vi "ClusterControls.vi"() -> ()   [LabVIEW 2016, in "test_ValueSignal.lvlib"]
uses:
  test_ValueSignal.lvlib
  Helper/HelperVI1.vi
  main/apis/Stimulus/ValueSignalByPathString.vi
  main/apis/Assert/AssertControlValueByPathString.vi
  <vilib>/addons/_JKI Toolkits/Caraya/classes/Assert/Assert Equal Value_Variant.vi
  <vilib>/addons/_JKI Toolkits/Caraya/classes/Assert/Assert.lvclass
  <vilib>/addons/_JKI Toolkits/Caraya/classes/Test/Test.lvclass
panel:
  out "error out":errorcluster
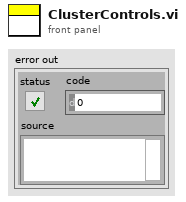
[diagram p1: front panel]
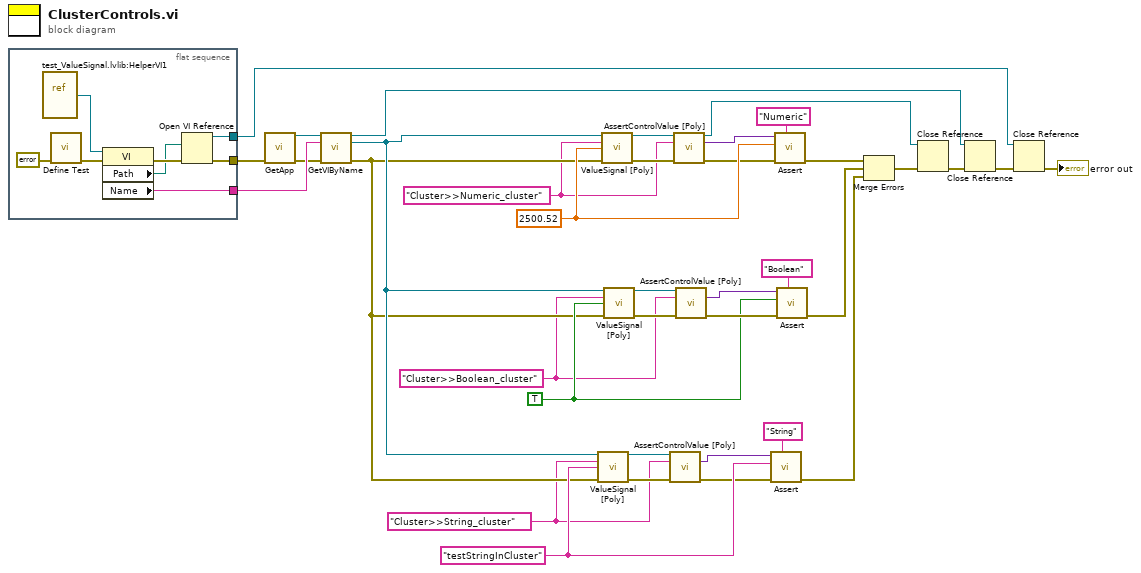
[diagram p0: block diagram]
diagram:
  w1 = "Cluster>>String_cluster"
  w2 = "Cluster>>Boolean_cluster"
  w3 = "Cluster>>Numeric_cluster"
  w17 = "testStringInCluster"
  w20 = TRUE
  w29 = 2500.52
  n1 = flat-sequence {
    tunnel: [w41] -> w32
    tunnel: [w40] -> w34
    tunnel: [w38] -> w31
    frame #0 {
      n2 = vi-ref "test_ValueSignal.lvlib:HelperVI1.vi"() -> (w43:refnum<vi>)
      n3 = call <vilib>:"Define Test.vi"("error in (no error)"=errorcluster {"status"=FALSE, "code"=0, "source"=""}) -> ("error out"=w44:errorcluster)  [unwired: 10 in]
      n4 = property on="Property Node" class="VI"(reference=w43, error in=w44) -> (error out=w42:errorcluster, "Path"=w39:path, "Name"=w38:string)  [unwired: 1 out]
      n5 = Open VI Reference(vi path=w39, error in (no error)=w42) -> (vi reference=w40:refnum<vi>, error out=w41:errorcluster)  [unwired: 4 in]
    }
  }
  n6 = call "GetApp.vi"("error in (no error)"=w32) -> ("Application Ref"=w33:refnum<vi>, "error out"=w30:errorcluster)  [unwired: 13 in]
  n7 = call "GetVIByName.vi"("Application Ref in"=w33, "VI Name"=w31, "error in (no error)"=w30) -> ("Application Ref out"=w5:refnum<vi>, "VI Reference"=w12:refnum<vi>, "error out"=w4:errorcluster)  [unwired: 10 in]
  n8 = call-poly "ValueSignal [Poly].vi"("VI Reference In"=w12, "Control Name"=w1, "Value (Signaling)"=w17, "error in"=w4) -> ("VI Reference Out"=w16:refnum<vi>, "error out"=w15:errorcluster)  [unwired: 10 in]
  n9 = call-poly "ValueSignal [Poly].vi"("VI Reference In"=w12, "Control Name"=w3, "Value (Signaling)"=w29, "error in"=w4) -> ("VI Reference Out"=w28:refnum<vi>, "error out"=w27:errorcluster)  [unwired: 10 in]
  n10 = call-poly "ValueSignal [Poly].vi"("VI Reference In"=w12, "Control Name"=w2, "Value (Signaling)"=w20, "error in"=w4) -> ("VI Reference Out"=w21:refnum<vi>, "error out"=w22:errorcluster)  [unwired: 10 in]
  n11 = call-poly "AssertControlValue [Poly].vi"("VI Reference In"=w16, "Control Name"=w1, "error in"=w15) -> ("Value"=w13:variant, "error out"=w14:errorcluster)  [unwired: 10 in, 1 out]
  n12 = call-poly "AssertControlValue [Poly].vi"("VI Reference In"=w28, "Control Name"=w3, "error in"=w27) -> ("VI Reference Out"=w7:refnum<vi>, "Value"=w25:variant, "error out"=w26:errorcluster)  [unwired: 10 in]
  n13 = call-poly "AssertControlValue [Poly].vi"("VI Reference In"=w21, "Control Name"=w2, "error in"=w22) -> ("Value"=w24:variant, "error out"=w23:errorcluster)  [unwired: 10 in, 1 out]
  n14 = call-poly <vilib>:"Assert.vi"("Label"="String" ("Label (VI Title)"), "error in (no error)"=w14, "Y"=w17, "X"=w13) -> ("error out"=w9:errorcluster)  [unwired: 7 in]
  n15 = call-poly <vilib>:"Assert.vi"("Label"="Numeric" ("Label (VI Title)"), "error in (no error)"=w26, "Y"=w29, "X"=w25) -> ("error out"=w36:errorcluster)  [unwired: 7 in]
  n16 = call-poly <vilib>:"Assert.vi"("Label"="Boolean" ("Label (VI Title)"), "error in (no error)"=w23, "Y"=w20, "X"=w24) -> ("error out"=w10:errorcluster)  [unwired: 7 in]
  n17 = Merge Errors(w36, w10, w9) -> (w11:errorcluster)
  n18 = Close Reference(reference=w7, error in (no error)=w11) -> (error out=w8:errorcluster)
  n19 = Close Reference(reference=w5, error in (no error)=w8) -> (error out=w6:errorcluster)
  n20 = Close Reference(reference=w34, error in (no error)=w6) -> (error out=→"error out":errorcluster)
